vi "Set Out.vi"(8 "error in":errorcluster, 11 "SL_SC in":refnum<class "SL_SC.lvclass">) -> (0 "error out":errorcluster, 3 "SL_SC out":refnum<class "SL_SC.lvclass">)   [LabVIEW 2019, in "SL_SC.lvlib" / "SL_SC.lvclass"]
uses:
  Library/SL_SC.lvclass
  C:/Users/Public/Documents/Development/builds/Instruments/DIG_IO.lvlibp/Library/DIG_IO.lvclass
  Library/SL_SC.lvclass/SL_SC.ctl
  builds/Instruments/DIG_IO.lvlibp/Accessors/Read Digital.vi
  <vilib>/SLSC/Set Device Property (U32).vi
  <vilib>/SLSC/Commit Properties for Devices.vi
  builds/Instruments/DIG_IO.lvlibp/Library/DIG_IO.lvclass
  <vilib>/SLSC/SLSC.lvlib
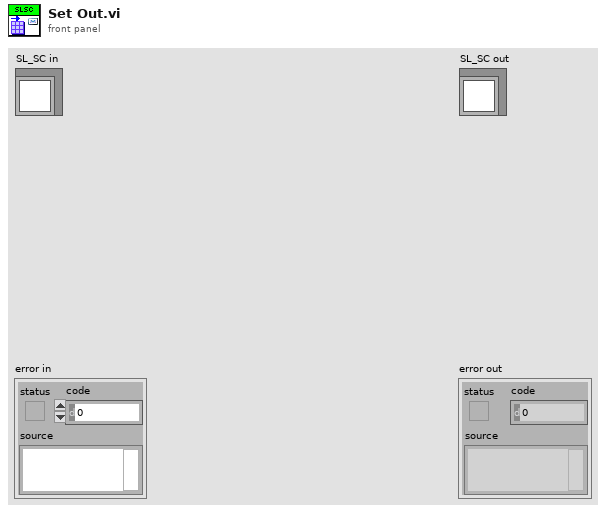
[diagram p1: front panel]
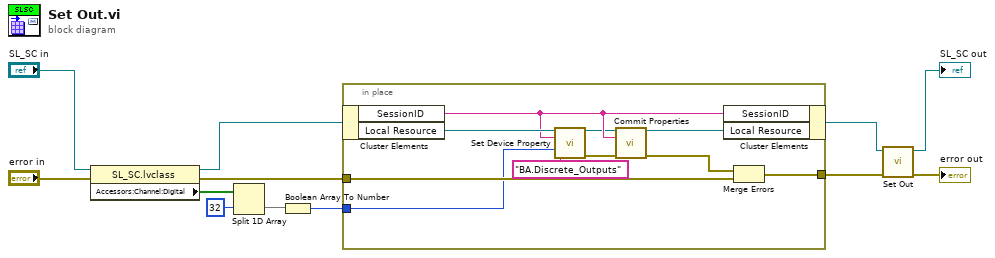
[diagram p0: block diagram]
diagram:
  n1 = property class="SL_SC.lvclass"(reference="SL_SC in", error in="error in") -> (reference out=w6:refnum<class "SL_SC.lvclass">, error out=w5:errorcluster, "Accessors:Channel:Digital"=w2:bool[])
  n2 = Split 1D Array(array=w2, index=32) -> (second subarray=w3:bool[])  [unwired: 1 out]
  n3 = Boolean Array To Number(Boolean array=w3) -> (number=w1:u32)
  n4 = in-place {
    in-place-border: w5 -> [w19]
    in-place-border: [w18] -> w7
    in-place-border: w1 -> [w14]
    n5 = in-place-cluster #1(w6) -> ("SessionID"=w21:string, "Local Resource"=w22:refnum<k21>)
    n6 = call-poly <vilib>:"Set Device Property.vi"("session in"=w22, "devices"=w21, "property"="BA.Discrete_Outputs", "property value"=w14) -> ("session out"=w16:refnum<k21>, "error out"=w15:errorcluster)  [unwired: 10 in]
    n7 = call-poly <vilib>:"Commit Properties.vi"("session in"=w16, "devices"=w21, "error in (no error)"=w15) -> ("session out"=w13:refnum<k21>, "error out"=w20:errorcluster)  [unwired: 11 in]
    n8 = in-place-cluster #1("SessionID"=w21, "Local Resource"=w13) -> (w8:refnum<class "SL_SC.lvclass">)
    n9 = Merge Errors(w20, w19) -> (w18:errorcluster)
  }
  n10 = call-parent "Set Out.vi"("error in"=w7, "DIG_IO in"=w8) -> ("error out"=→"error out":errorcluster, "DIG_IO out"=→"SL_SC out":refnum<class "SL_SC.lvclass">)  [unwired: 8 in]
